vi "Count Adjacent Black Tiles.vi"(10 "Current Tile":cluster{"x":i32, "y":i32, "z":i32}, 11 "Black Tiles":set{cluster{"x":i32, "y":i32, "z":i32}}(c389)) -> (2 "Black Neighbours":i16)   [LabVIEW 2020]
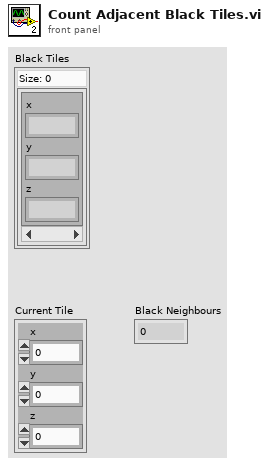
[diagram p1: front panel]
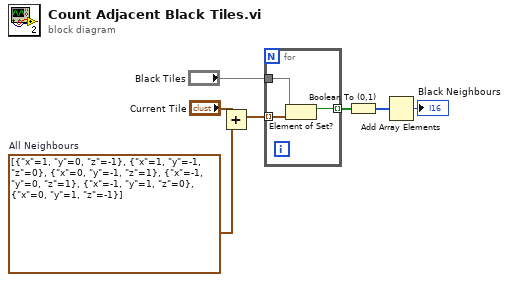
[diagram p0: block diagram]
diagram:
  w1 = cluster{"x":i32, "y":i32, "z":i32}[] [{"x"=1, "y"=0, "z"=-1}, {"x"=1, "y"=-1, "z"=0}, {"x"=0, "y"=-1, "z"=1}, {"x"=-1, "y"=0, "z"=1}, {"x"=-1, "y"=1, "z"=0}, {"x"=0, "y"=1, "z"=-1}]  # All Neighbours
  n1 = Add(x="Current Tile", y=w1) -> (x+y=w3:cluster{"x":i32, "y":i32, "z":i32}[])
  n2 = for {
    tunnel: w3 -> [w10] mode=indexing
    tunnel: [w8] -> w4 mode=indexing
    tunnel: "Black Tiles" -> [w9]
    n3 = Element of Set?(10:w10, 11:w9) -> (3:w8:bool)
  }
  n4 = Boolean To (0,1)(Boolean=w4) -> (0, 1=w5:i16[])
  n5 = Add Array Elements(numeric array=w5) -> (sum=→"Black Neighbours":i16)
